vi "edit-data.vi"(10 "Hardware Resources in":T1={"DAQmx Channel 1"="", "DAQmx Channel 2"="", "DAQmx Channel 3"="", "Channel 1 Name"="", "Channel 2 Name"="", "Channel 3 Name"="", "Input Config Channel 1"=-1, "Input Config Channel 2"=-1, "Input Config Channel 3"=-1, "Offset Channel 1"=0.0, "Offset Channel 2"=0.0, "Offset Channel 3"=0.0, "Scale Channel 1"=0.0, "Scale Channel 2"=0.0, "Scale Channel 3"=0.0, "Sample time"=0, "Samples per second"=0.0, "Sample mode"=0, "Samples per channel"=0, "DAQmx AI Task"="", "DAQmx Channel 4"="", "Channel 3 Name 2"="", "Input Config Channel 4"=-1, "Offset Channel 4"=0.0, "Scale Channel 4"=0.0} {"Input Config Channel 4" items=["Default"=-1, "RSE"=10083, "NRSE"=10078, "Differential"=10106, "Pseudodifferential"=12529]; "Input Config Channel 3" items=["Default"=-1, "RSE"=10083, "NRSE"=10078, "Differential"=10106, "Pseudodifferential"=12529]; "Input Config Channel 2" items=["Default"=-1, "RSE"=10083, "NRSE"=10078, "Differential"=10106, "Pseudodifferential"=12529]; "Input Config Channel 1" items=["Default"=-1, "RSE"=10083, "NRSE"=10078, "Differential"=10106, "Pseudodifferential"=12529]; "Sample mode" items=["Hardware Timed Single Point"=12522, "Finite Samples"=10178, "Continuous Samples"=10123]}, 11 "data":waveform(dbl)[](array[waveform])) -> (3 "Array of Waveform":waveform(dbl)[](array[waveform]))   [LabVIEW 2018, in "Acquisition.lvlib"]
uses:
  Acquisition.lvlib
  Hardware Configuration.ctl
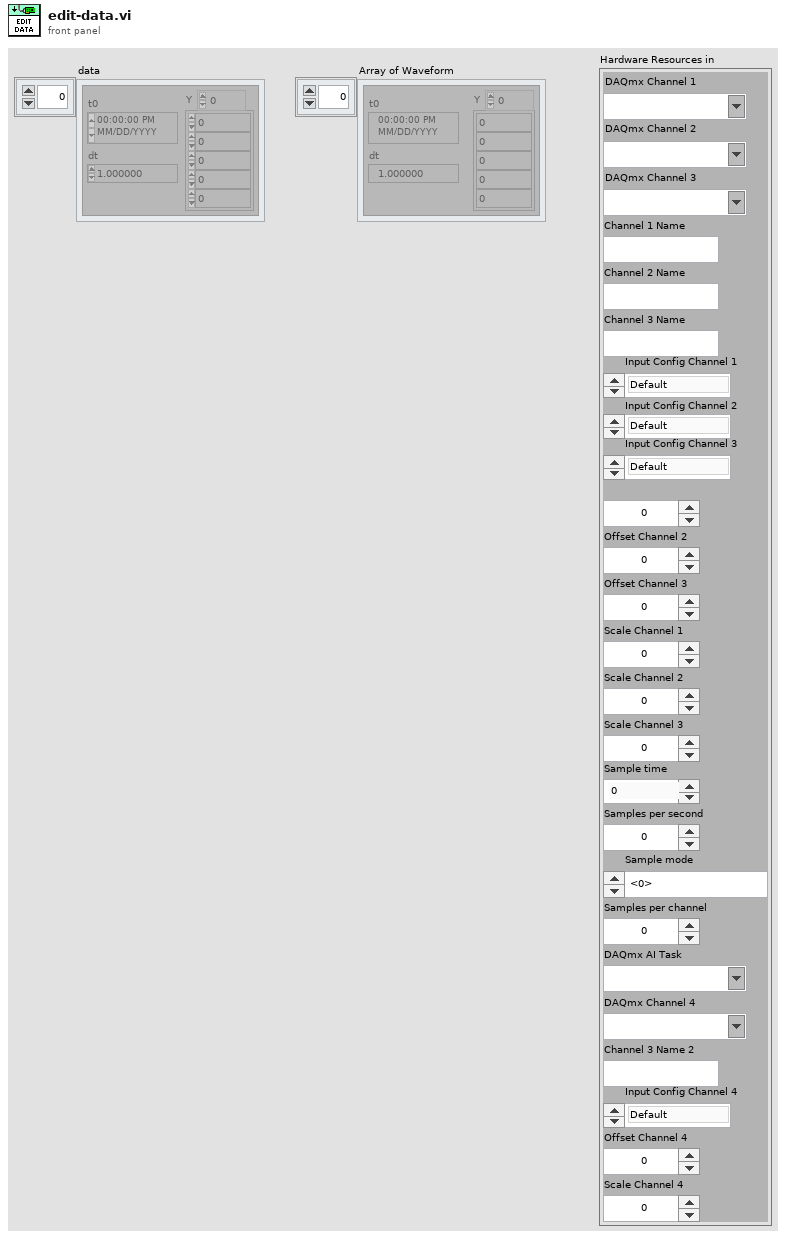
[diagram p1: front panel]
types:
  T1 = typedef "Acquisition.lvlib/Hardware Configuration.ctl" = cluster{"DAQmx Channel 1":tag, "DAQmx Channel 2":tag, "DAQmx Channel 3":tag, "Channel 1 Name":string, "Channel 2 Name":string, "Channel 3 Name":string, "Input Config Channel 1":i32, "Input Config Channel 2":i32, "Input Config Channel 3":i32, "Offset Channel 1":dbl, "Offset Channel 2":dbl, "Offset Channel 3":dbl, "Scale Channel 1":dbl, "Scale Channel 2":dbl, "Scale Channel 3":dbl, "Sample time":u32, "Samples per second":dbl, "Sample mode":u16, "Samples per channel":i32, "DAQmx AI Task":refnum<k21>, "DAQmx Channel 4":tag, "Channel 3 Name 2":string, "Input Config Channel 4":i32, "Offset Channel 4":dbl, "Scale Channel 4":dbl}
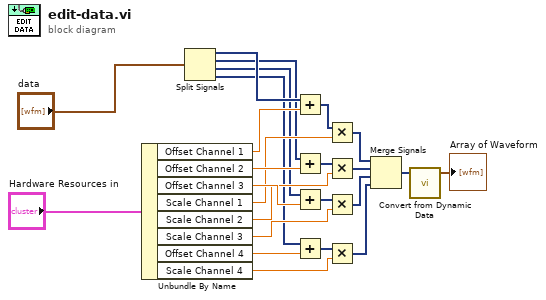
[diagram p0: block diagram]
diagram:
  n1 = Unbundle By Name("Hardware Resources in") -> ("Offset Channel 1"=w19:dbl, "Offset Channel 2"=w21:dbl, "Offset Channel 3"=w23:dbl, "Scale Channel 1"=w20:dbl, "Scale Channel 2"=w22:dbl, "Scale Channel 3"=w24:dbl, "Offset Channel 4"=w4:dbl, "Scale Channel 4"=w3:dbl)
  n2 = Split Signals("data") -> (w8:dynamicdata, w7:dynamicdata, w6:dynamicdata, w1:dynamicdata)  [unwired: 4 in]
  n3 = Add(x=w8, y=w19) -> (x+y=w10:dynamicdata)
  n4 = Add(x=w7, y=w21) -> (x+y=w11:dynamicdata)
  n5 = Add(x=w6, y=w23) -> (x+y=w12:dynamicdata)
  n6 = Add(x=w1, y=w4) -> (x+y=w5:dynamicdata)
  n7 = Multiply(x=w10, y=w20) -> (x*y=w13:dynamicdata)
  n8 = Multiply(x=w11, y=w22) -> (x*y=w14:dynamicdata)
  n9 = Multiply(x=w12, y=w24) -> (x*y=w15:dynamicdata)
  n10 = Multiply(x=w5, y=w3) -> (x*y=w2:dynamicdata)
  n11 = Merge Signals(w13, w14, w15, w2) -> (w16:dynamicdata)
  n12 = call "Convert from Dynamic Data"("Dynamic Data Type"=w16) -> ("Array of Waveform"=→"Array of Waveform":waveform(dbl)[])  [unwired: 3 in]
